vi "NewDataEvent.vi"(8 "error in (no error)":errorcluster, 9 "data flow":T17, 10 "data event config":T6, 11 "config":T16) -> (0 "error out":errorcluster, 2 "data event config":T6, 3 "data event":T9, 4 "registry":T1, 5 "save waveforms":bool)   [LabVIEW 2017, in "EmsaDataEventCreator.lvlib"]
uses:
  <vilib>/addons/InsightCM/Devices/Shared/Emsa/EmsaDataEventCreator/EmsaDataEventCreator.lvlib
  <vilib>/addons/InsightCM/Devices/Shared/Common/DataFlow/controls/Data.ctl
  <vilib>/addons/InsightCM/Utilities/DataAccessors/controls/wfmSGL_DVR.ctl
  <vilib>/addons/PointValueMap/controls/PointMap.ctl
  <vilib>/addons/InsightCM/Devices/Shared/Common/DataFlow/controls/Type.ctl
  <vilib>/addons/InsightCM/Devices/Shared/Emsa/EmsaDataEventCreator/controls/DataEventConfig.ctl
  <vilib>/addons/InsightCM/Devices/Shared/Emsa/EmsaDataEventCreator/controls/SweepParams.ctl
  <vilib>/addons/InsightCM/Devices/Shared/Emsa/EmsaDataEventCreator/controls/config.ctl
  <vilib>/addons/InsightCM/Devices/Shared/Common/DataEvent/controls/Event.ctl
  <vilib>/addons/InsightCM/MessageBus/Base/controls/DataEvent.ctl
  <vilib>/addons/InsightCM/MessageBus/Base/controls/KeyValuePair.ctl
  <vilib>/addons/InsightCM/Devices/Shared/Common/DataEvent/controls/DataSet.ctl
  <vilib>/addons/InsightCM/MessageBus/Base/controls/DataSetMetadata.ctl
  <vilib>/addons/InsightCM/MessageBus/Base/controls/TrendPoint.ctl
  <vilib>/addons/InsightCM/MessageBus/Base/controls/TrendAlarmUpdate.ctl
  <vilib>/addons/InsightCM/MessageBus/Base/controls/TrendAlarmTransition.ctl
  <vilib>/addons/InsightCM/Devices/Shared/Emsa/EmsaDataEventCreator/controls/Registry.ctl
  <vilib>/addons/InsightCM/Devices/Shared/Emsa/EmsaDataEventCreator/controls/Registry_Sweep.ctl
  <vilib>/addons/InsightCM/Devices/Shared/Common/DataEvent/controls/DataSetType.ctl
  <vilib>/addons/InsightCM/Devices/Shared/Common/DataEventCreator/controls/Registry_Trend.ctl
  <vilib>/addons/InsightCM/Devices/Shared/Common/DataEvent/DataEvent.lvlib
  <vilib>/addons/InsightCM/SRP/SRP.lvlib
  <vilib>/addons/InsightCM/Devices/Shared/Common/DataEventCreator/DataEventCreator.lvlib
  <vilib>/addons/PointValueMap/PointValueMap.lvlib
  <vilib>/addons/InsightCM/Devices/Shared/Common/DataFlow/DataFlow.lvlib
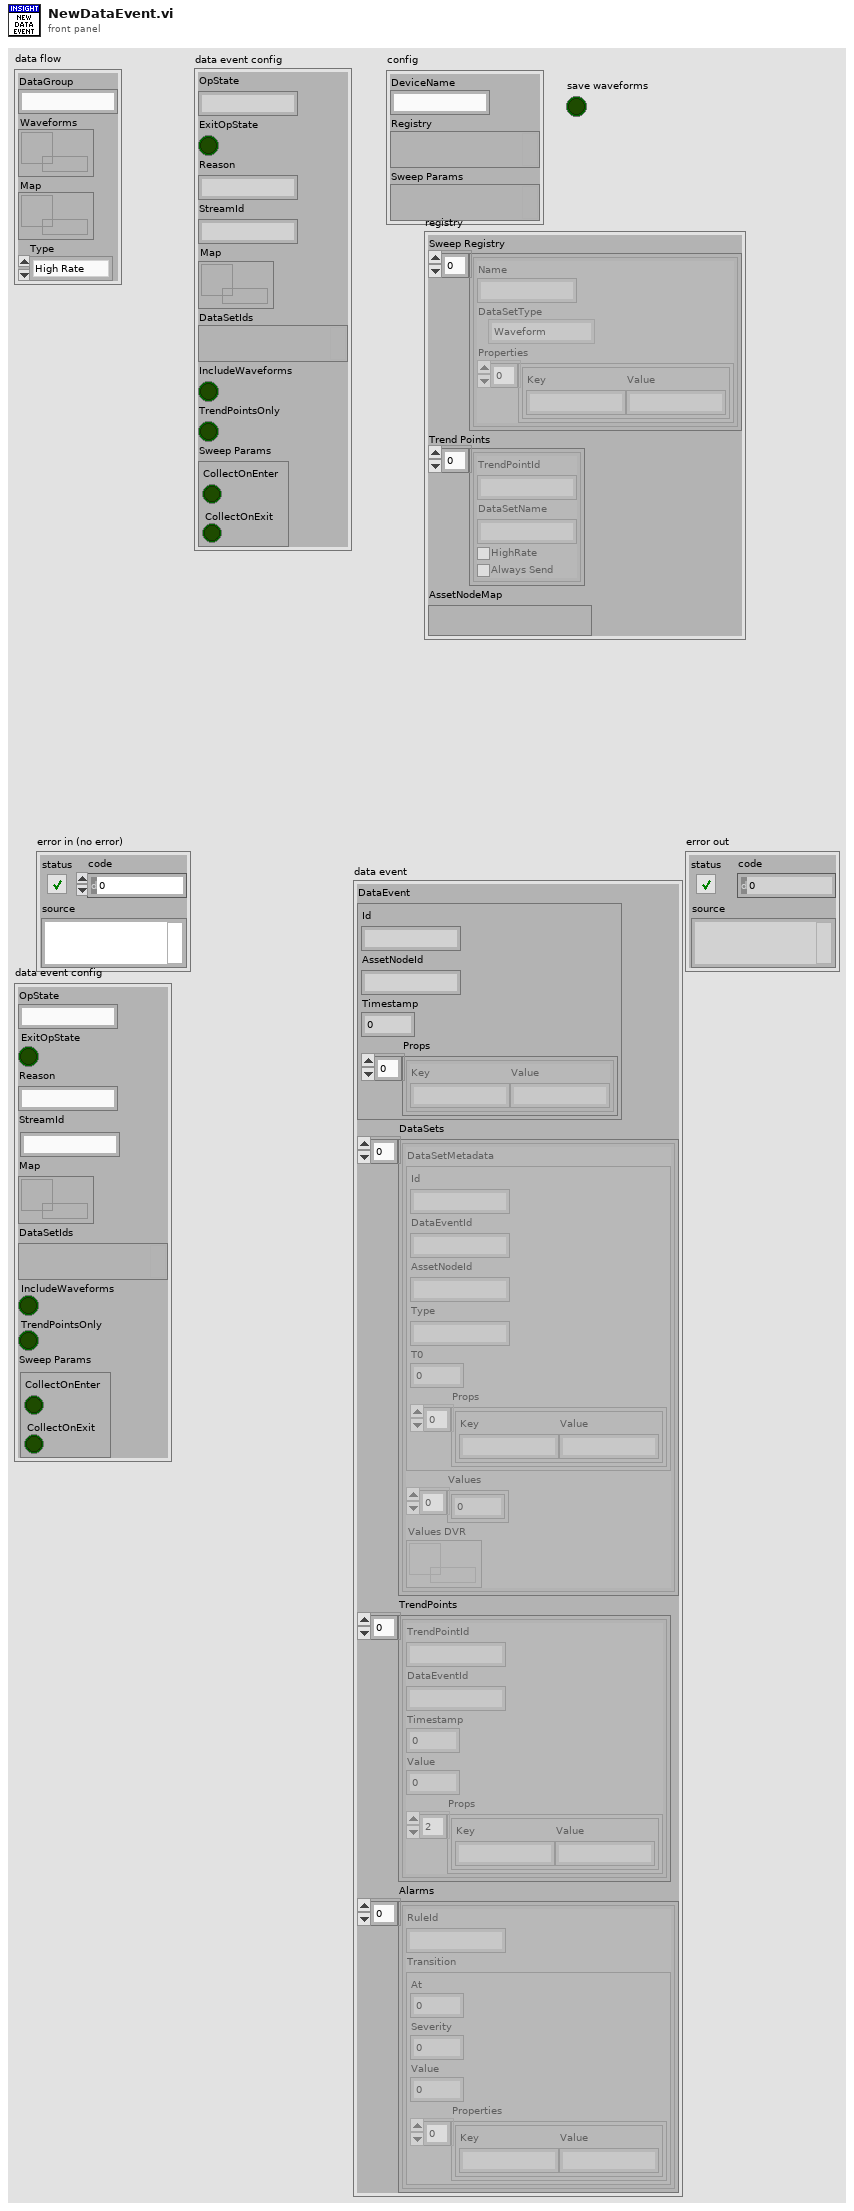
[diagram p1: front panel]
types:
  T1 = typedef "EmsaDataEventCreator.lvlib/Registry.ctl" = cluster{"Sweep Registry":T2[], "Trend Points":T5[], "AssetNodeMap":variant}
  T2 = typedef "EmsaDataEventCreator.lvlib/Registry_Sweep.ctl" = cluster{"Name":string, "DataSetType":T3, "Properties":T4[]}
  T3 = typedef "DataEvent.lvlib/DataSetType.ctl" = enum16{"Waveform", "SpeedProfile", "ThermalImage", "EmsaSweep"}
  T4 = typedef "KeyValuePair.ctl" = cluster{"Key":string, "Value":string}
  T5 = typedef "DataEventCreator.lvlib/Registry_Trend.ctl" = cluster{"TrendPointId":string, "DataSetName":string, "HighRate":bool, "Always Send":bool}
  T6 = typedef "EmsaDataEventCreator.lvlib/DataEventConfig.ctl" = cluster{"OpState":string, "ExitOpState":bool, "Reason":string, "StreamId":string, "Map":T7, "DataSetIds":variant, "IncludeWaveforms":bool, "TrendPointsOnly":bool, "Sweep Params":T8}
  T7 = typedef "PointValueMap.lvlib/PointMap.ctl" = refnum<data-value>
  T8 = typedef "EmsaDataEventCreator.lvlib/SweepParams.ctl" = cluster{"CollectOnEnter":bool, "CollectOnExit":bool}
  T9 = typedef "DataEvent.lvlib/Event.ctl" = cluster{"DataEvent":T10, "DataSets":T11[], "TrendPoints":T13[], "Alarms":T14[]}
  T10 = typedef "DataEvent.ctl" = cluster{"Id":string, "AssetNodeId":string, "Timestamp":i64, "Props":T4[]}
  T11 = typedef "DataEvent.lvlib/DataSet.ctl" = cluster{"DataSetMetadata":T12, "Values":sgl[], "Values DVR":refnum<data-value>}
  T12 = typedef "DataSetMetadata.ctl" = cluster{"Id":string, "DataEventId":string, "AssetNodeId":string, "Type":string, "T0":i64, "Props":T4[]}
  T13 = typedef "TrendPoint.ctl" = cluster{"TrendPointId":string, "DataEventId":string, "Timestamp":i64, "Value":dbl, "Props":T4[]}
  T14 = typedef "TrendAlarmUpdate.ctl" = cluster{"RuleId":string, "Transition":T15}
  T15 = typedef "TrendAlarmTransition.ctl" = cluster{"At":i64, "Severity":i32, "Value":dbl, "Properties":T4[]}
  T16 = typedef "EmsaDataEventCreator.lvlib/config.ctl" = cluster{"DeviceName":string, "Registry":variant, "Sweep Params":variant}
  T17 = typedef "DataFlow.lvlib/Data.ctl" = cluster{"DataGroup":string, "Waveforms":T18, "Map":T7, "Type":T19}
  T18 = typedef "wfmSGL_DVR.ctl" = refnum<data-value>
  T19 = typedef "DataFlow.lvlib/Type.ctl" = enum16{"High Rate", "Low Rate", "Burst Mode"}
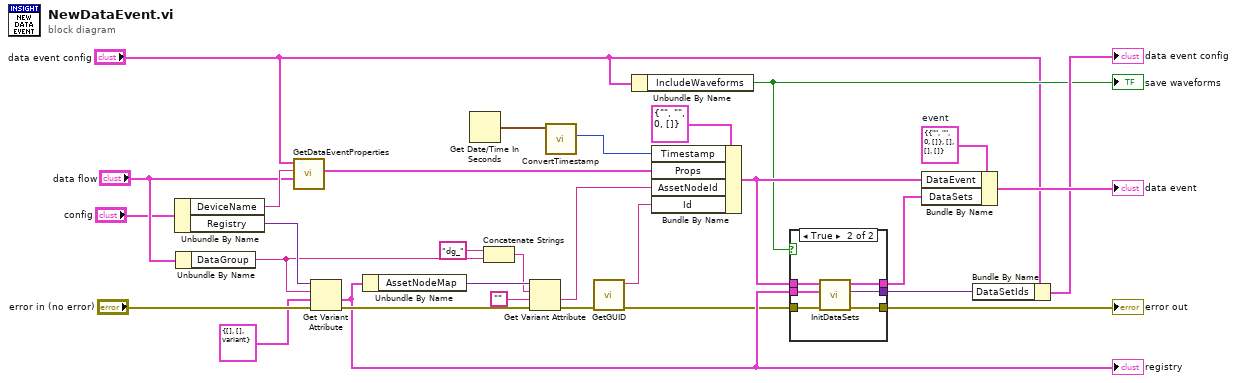
[diagram p0: block diagram]
diagram:
  w29 = T9 {"DataEvent"={"Id"="", "AssetNodeId"="", "Timestamp"=0, "Props"=[]}, "DataSets"=[], "TrendPoints"=[], "Alarms"=[]}  # event
  n1 = Unbundle By Name("config") -> ("DeviceName"=w19:string, "Registry"=w30:variant)
  n2 = Unbundle By Name("data flow") -> ("DataGroup"=w2:string)
  n3 = call <vilib>:"GetDataEventProperties.vi"("data"="data flow", "device name"=w19, "data event config"="data event config") -> ("data event properties"=w20:T4[])  [unwired: 8 in]
  n4 = Get Variant Attribute(Variant=w30, name=w2, default value (empty Variant)=T1 {"Sweep Registry"=[], "Trend Points"=[], "AssetNodeMap"=variant} ("Registry"), error in="error in (no error)") -> (value=w17:T1, error out=w26:errorcluster)  [unwired: 2 out]
  "registry" <- w17
  n5 = Unbundle By Name(w17) -> ("AssetNodeMap"=w27:variant)
  n6 = Get Date/Time In Seconds() -> (seconds since 1Jan1904=w8:timestamp)
  n7 = Concatenate Strings("dg_" ("string"), w2) -> (w1:string)
  n8 = Get Variant Attribute(Variant=w27, name=w1, default value (empty Variant)="", error in=w26) -> (value=w24:string, error out=w21:errorcluster)  [unwired: 2 out]
  n9 = call <vilib>:"ConvertTimestamp.vi"("Time Stamp"=w8) -> ("Timestamp out"=w7:i64)  [unwired: 10 in]
  n10 = call <vilib>:"GetGUID.vi"("error in (no error)"=w21) -> ("error out"=w16:errorcluster, "GUID"=w23:string)  [unwired: 9 in]
  n11 = Unbundle By Name("data event config") -> ("IncludeWaveforms"=w6:bool)
  "save waveforms" <- w6
  n12 = Bundle By Name(cluster=T10 {"Id"="", "AssetNodeId"="", "Timestamp"=0, "Props"=[]} ("DataEvent"), "Timestamp"=w7, "Props"=w20, "AssetNodeId"=w24, "Id"=w23) -> (w13:T10)
  n13 = case shown="True" w6 {
    tunnel: w17 -> [_ w33]
    tunnel: w16 -> [w31 w37]
    tunnel: [_ w36] -> w15
    tunnel: [w31 w35] -> w10
    tunnel: [_ w34] -> w14
    tunnel: w13 -> [_ w32]
    frame False {
    }
    frame True {
      n14 = call <vilib>:"InitDataSets.vi"("error in (no error)"=w37, "registry"=w33, "dataevent"=w32) -> ("error out"=w35:errorcluster, "datasetIds"=w36:variant, "datasets"=w34:T11[])  [unwired: 6 in]
    }
  }
  "error out" <- w10
  n15 = Bundle By Name(cluster=w29, "DataEvent"=w13, "DataSets"=w14) -> (→"data event":T9)
  n16 = Bundle By Name(cluster="data event config", "DataSetIds"=w15) -> (→"data event config":T6)
